vi "TCP Named Service - Client.vi"() -> ()   [LabVIEW 2014]
doc: "This VI implements a client for the TCP Named Service - Server.vi. It connects to a service by specifying the server address and the name of the service. The client receives the string sent by the server, displays the string and closes the connection."
panel:
  in  "data in":string="Received"
  out "Message from Server":string
  # "Overview: Demonstrates the use of the TCP functions to connect to a TCP server VI via named service and receive data.\nInstructions:\n1. Ensure TCP Named Service - Server.vi is already running.\n2. Run the VI."
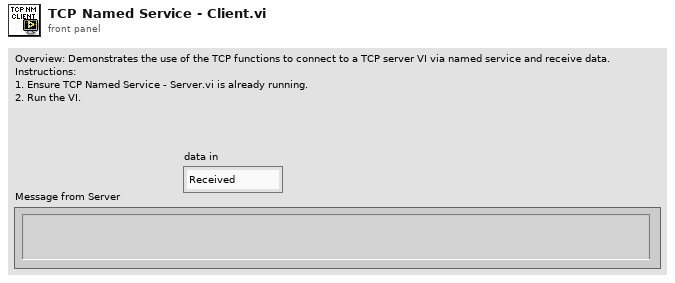
[diagram p1: front panel]
types:
  T1 = enum16{"Standard", "Buffered", "CRLF", "Immediate"}
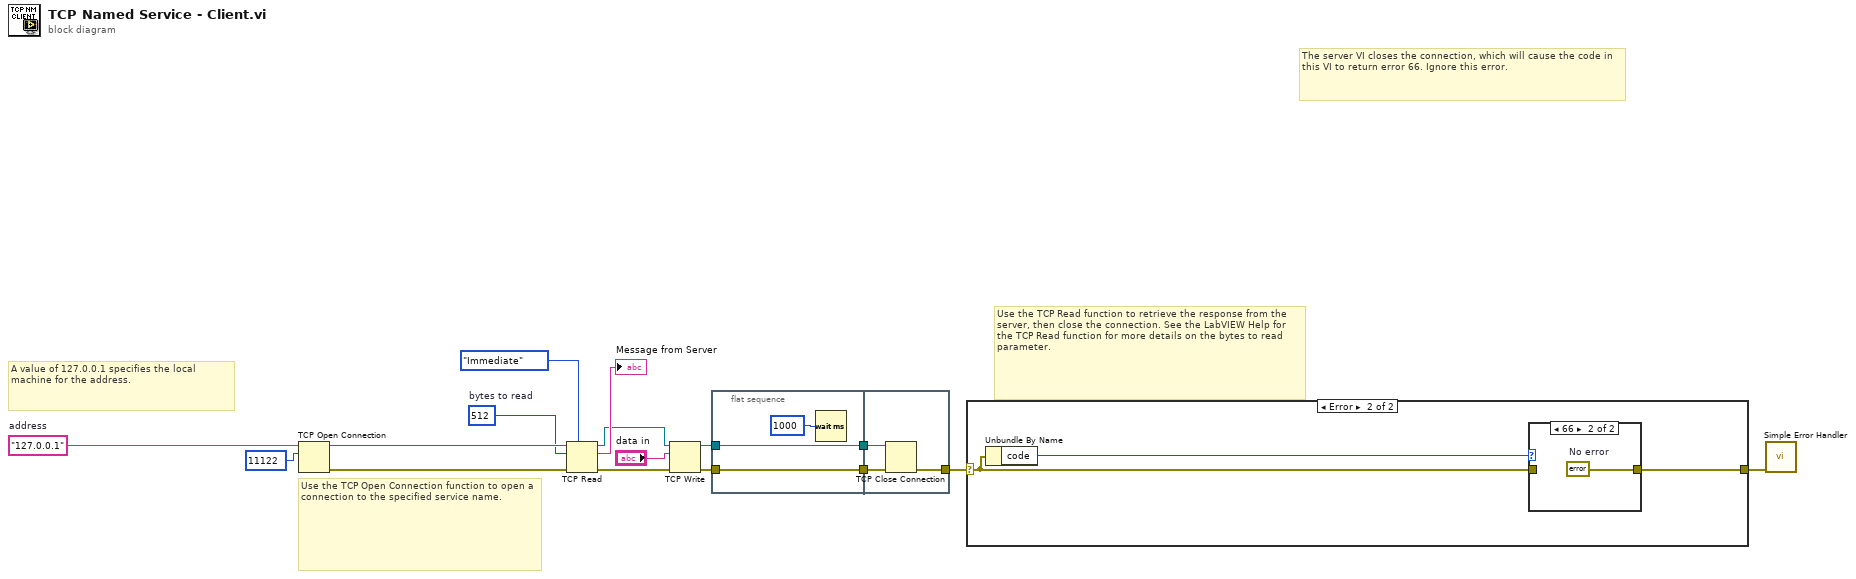
[diagram p0: block diagram]
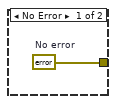
[diagram p2: hidden frame]
diagram:
  w12 = 512  # bytes to read
  w13 = "127.0.0.1"  # address
  # "The server VI closes the connection, which will cause the code in this VI to return error 66. Ignore this error."
  # "A value of 127.0.0.1 specifies the local machine for the address."
  # "Use the TCP Open Connection function to open a connection to the specified service name."
  # "Use the TCP Read function to retrieve the response from the server, then close the connection. See the LabVIEW Help for the TCP Read function for more details on the bytes to read parameter."
  n1 = TCP Open Connection(address=w13, remote port or service name=u16 11122) -> (connection ID=w15:refnum<k5>, error out=w16:errorcluster)  [unwired: 3 in]
  n2 = TCP Read(connection ID=w15, bytes to read=w12, error in (no error)=w16, 7:T1."Immediate" ("mode (standard)")) -> (connection ID out=w5:refnum<k5>, data out=→"Message from Server":string, error out=w7:errorcluster)  [unwired: 1 in]
  n3 = TCP Write(connection ID=w5, data in="data in", error in (no error)=w7) -> (connection ID out=w6:refnum<k5>, error out=w8:errorcluster)  [unwired: 1 in, 1 out]
  n4 = flat-sequence {
    tunnel: w6 -> [w18]
    tunnel: w8 -> [w19]
    tunnel: [w19] -> w2
    tunnel: [w18] -> w1
    tunnel: [w22] -> w11
    tunnel: w2 -> [w21]
    tunnel: w1 -> [w20]
    frame #0 {
      n5 = Wait (ms)(milliseconds to wait=u32 1000) -> ()  [unwired: 1 out]
    }
    frame #1 {
      n6 = TCP Close Connection(connection ID=w20, error in (no error)=w21) -> (error out=w22:errorcluster)  [unwired: 1 in, 1 out]
    }
  }
  n7 = case shown="Error" w11 {
    selector: w11 -> [_ w25]
    tunnel: [w23 w24] -> w10
    frame No Error {
      w23 = errorcluster {"status"=FALSE, "code"=0, "source"=""}  # No error
    }
    frame Error {
      n8 = Unbundle By Name(w25) -> ("code"=w26:i32)
      n9 = case shown="66" w26 {
        tunnel: w25 -> [w27 _]
        tunnel: [w27 w28] -> w24
        frame Default {
        }
        frame 66 {
          w28 = errorcluster {"status"=FALSE, "code"=0, "source"=""}  # No error
        }
      }
    }
  }
  n10 = call <vilib>:"Simple Error Handler.vi"("error in (no error)"=w10) -> ()  [unwired: 4 in, 5 out]
